vi "Emergency Stop.vi"(8 "error in":errorcluster) -> (0 "error out":errorcluster, 2 "Stage current position":dbl[](array[numeric]))   [LabVIEW 2017]
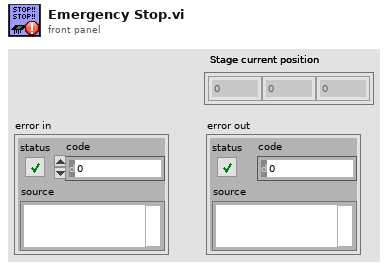
[diagram p1: front panel]
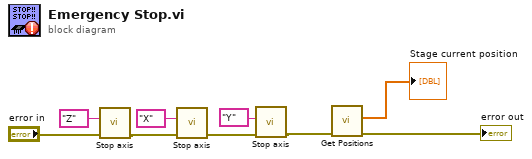
[diagram p0: block diagram]
diagram:
  n1 = call "Stop axis.vi"("error in"="error in", "Axis to stop"="Z") -> ("error out"=w3:errorcluster)  [unwired: 9 in]
  n2 = call "Stop axis.vi"("error in"=w3, "Axis to stop"="X") -> ("error out"=w2:errorcluster)  [unwired: 9 in]
  n3 = call "Stop axis.vi"("error in"=w2, "Axis to stop"="Y") -> ("error out"=w7:errorcluster)  [unwired: 9 in]
  n4 = call "Get Positions.vi"("error in"=w7) -> ("error out"=→"error out":errorcluster, "Stage current position"=→"Stage current position":dbl[])  [unwired: 9 in]
